vi "LinearSystemLoop_GetXHat.vi"(11 "input inear System Loop":T1) -> (3 "XHat":T3)   [LabVIEW 2019, in "Trajectory_Library.lvlib"]
doc: "Returns the observer's state estimate x-hat.\n \nInputs:\n - LinearSystemLoop -- system data cluster\n\nOutputs:\n - XHat -- the observer's state estimate x-hat."
uses:
  Trajectory_Library.lvlib
  TypeDef/LINEAR_SYSTEM.ctl
  <vilib>/Analysis/Matrix/Datatypes/RealMatrix.ctl
  <vilib>/Analysis/Matrix/NI_Matrix.lvlib
  TypeDef/LINEAR_QUADRATIC_REGULATOR.ctl
  TypeDef/LINEAR_PLANT_INV_FF.ctl
  TypeDef/KALMAN_FILTER.ctl
  TypeDef/LINEAR_SYSTEM_LOOP.ctl
panel:
  # "<States,1>"
  # "<FUTURE --- CLAMP TYPE -- For now\nuse Normalize>"
  # "Steady State Gain  \n<States,Outputs>"
  # "State Estimate <Statess,1>"
  # "<States,States>"
  # "<States,Inputs>"
  # "<Outputs,States>"
  # "<Outputs,Inputs>"
  # "<States,1>"
  # "<Inputs,1>"
  # "<States,Inputs>"
  # "<States,States>"
  # "Ref State <States,1>"
  # "Comp and capped \noutput <Inputs,1>"
  # "Controller gain\n<Inputs,States>"
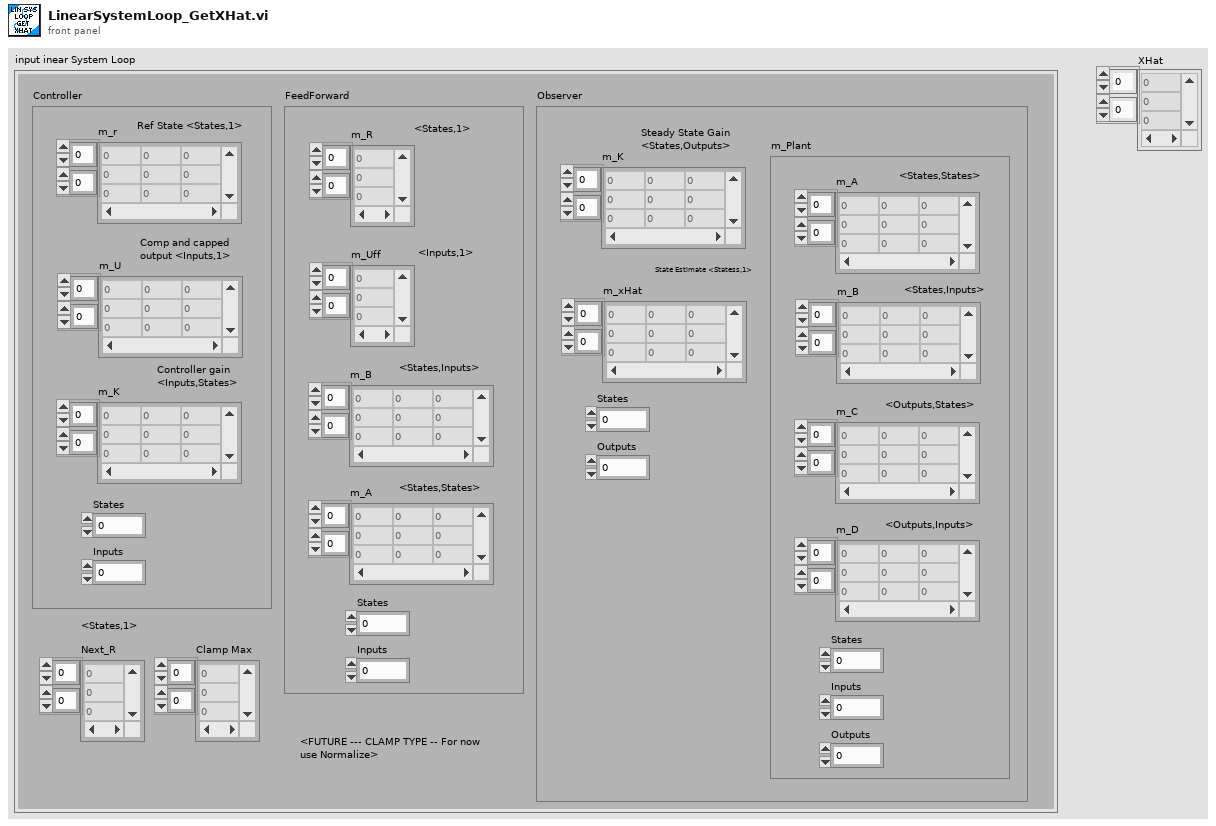
[diagram p1: front panel]
types:
  T1 = typedef "Trajectory_Library.lvlib/LINEAR_SYSTEM_LOOP.ctl" = cluster{"Controller":T2, "FeedForward":T4, "Observer":T5, "Next_R":T3, "Clamp Max":T3}
  T2 = typedef "Trajectory_Library.lvlib/LINEAR_QUADRATIC_REGULATOR.ctl" = cluster{"m_r":T3, "m_U":T3, "m_K":T3, "States":i32, "Inputs":i32}
  T3 = typedef "NI_Matrix.lvlib/RealMatrix.ctl" = dbl[][]
  T4 = typedef "Trajectory_Library.lvlib/LINEAR_PLANT_INV_FF.ctl" = cluster{"m_R":T3, "m_Uff":T3, "m_B":T3, "m_A":T3, "States":i32, "Inputs":i32}
  T5 = typedef "Trajectory_Library.lvlib/KALMAN_FILTER.ctl" = cluster{"m_K":T3, "m_xHat":T3, "States":i32, "Outputs":i32, "m_Plant":T6}
  T6 = typedef "Trajectory_Library.lvlib/LINEAR_SYSTEM.ctl" = cluster{"m_A":T3, "m_B":T3, "m_C":T3, "m_D":T3, "States":i32, "Inputs":i32, "Outputs":i32}
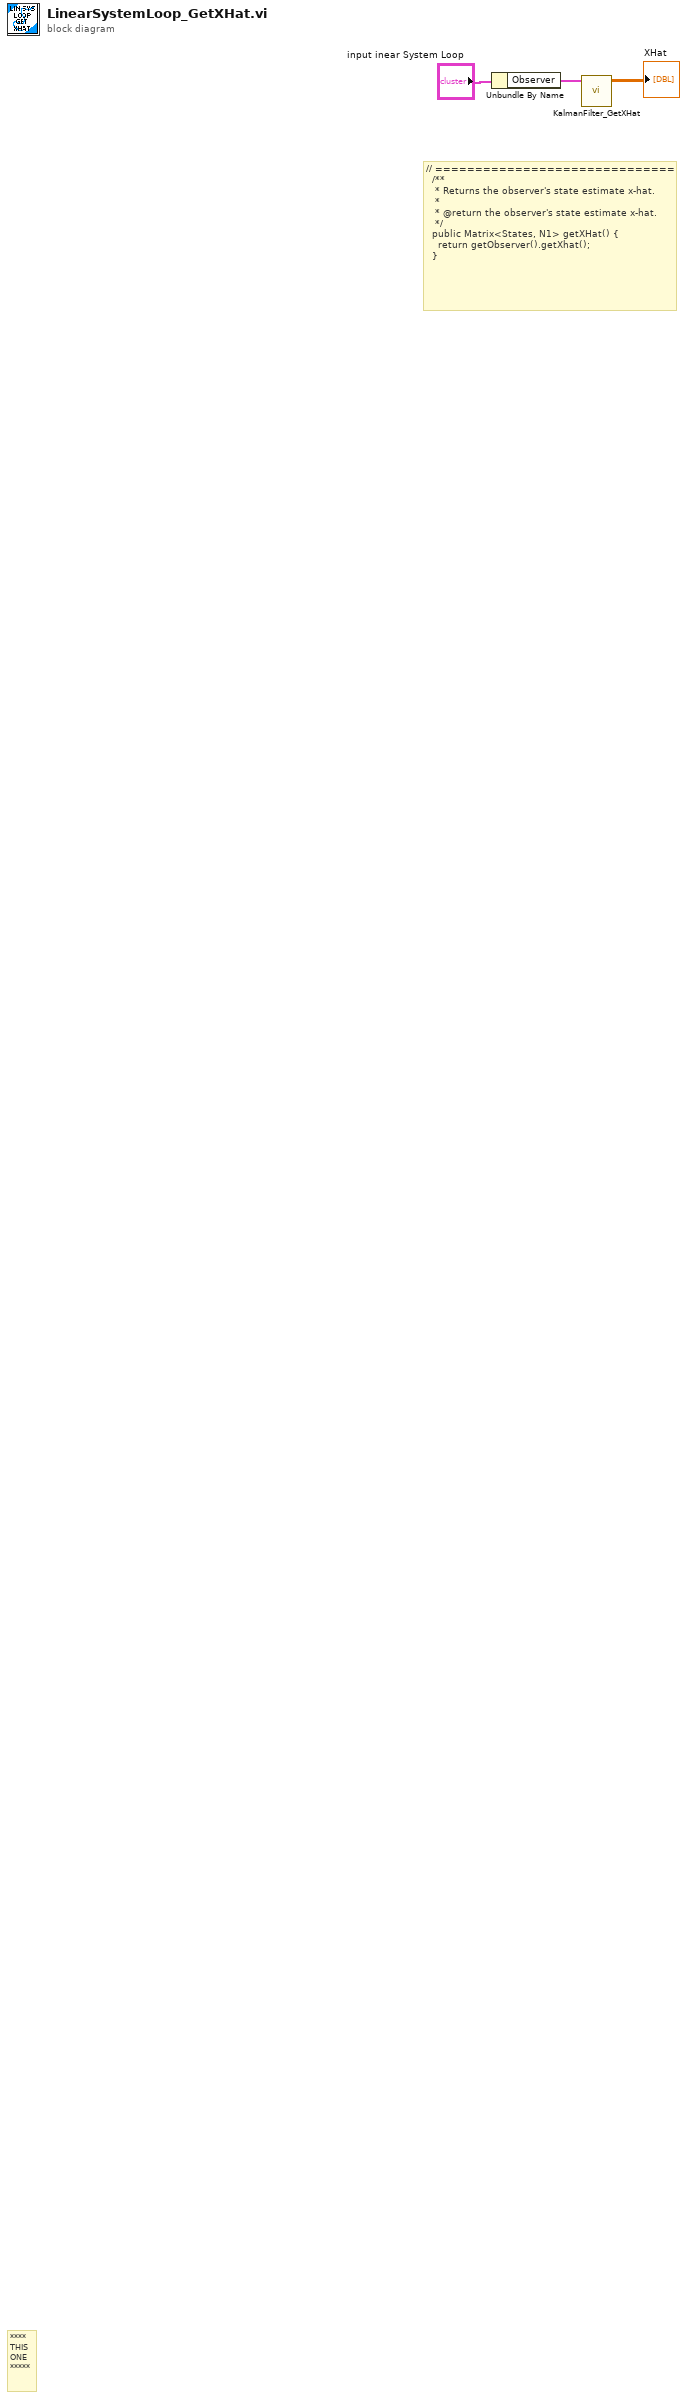
[diagram p0: block diagram]
diagram:
  # "// ==============================\n  /**\n   * Returns the observer's state estimate x-hat.\n   *\n   * @return the observer's state estimate x-hat.\n   */\n  public Matrix<States, N1> getXHat() {\n    return getObserver().getXhat();\n  }"
  # "****\nTHIS\nONE\n*****"
  n1 = Unbundle By Name("input inear System Loop") -> ("Observer"=w2:T5)
  n2 = call "KalmanFilter_GetXHat.vi"("in KalmanFilter"=w2) -> ("xHat"=→"XHat":T3)  [unwired: 10 in]
